vi "timer.vi"(8 "time in [ms]":u32, 11 "error in (no error)":errorcluster) -> (0 "time out [ms]":u32, 3 "error out":errorcluster, 4 "time difference [ms]":u32)   [LabVIEW 2013]
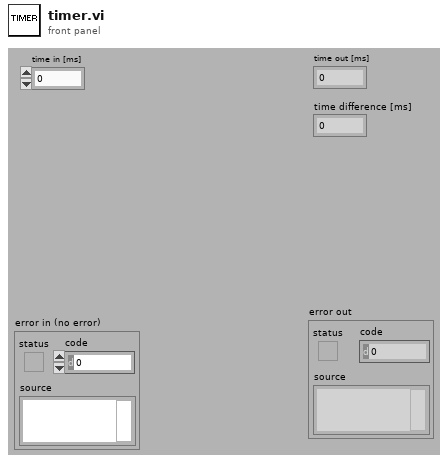
[diagram p1: front panel]
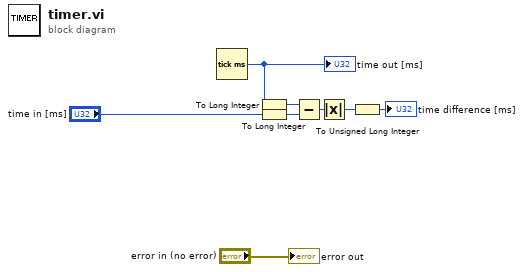
[diagram p0: block diagram]
diagram:
  n1 = Tick Count (ms)() -> (millisecond timer value=w7:u32)
  "time out [ms]" <- w7
  n2 = To Long Integer(number=w7) -> (32bit integer=w5:i32)
  n3 = To Long Integer(number="time in [ms]") -> (32bit integer=w4:i32)
  n4 = Subtract(x=w5, y=w4) -> (x-y=w3:i32)
  n5 = Absolute Value(x=w3) -> (abs(x)=w2:i32)
  n6 = To Unsigned Long Integer(number=w2) -> (unsigned 32bit integer=→"time difference [ms]":u32)
  "error out" <- "error in (no error)"
